vi "close buffer.vi"(8 "error in (no error)":errorcluster, 11 "Data Buffer in":refnum<class "Data Buffer.lvclass">) -> (0 "error out":errorcluster, 3 "Data Buffer out":refnum<class "Data Buffer.lvclass">)   [LabVIEW 2022 SP3, in "Data Buffer.lvclass"]
uses:
  Data Buffer.lvclass
  Data Buffer.lvclass/Data Buffer.ctl
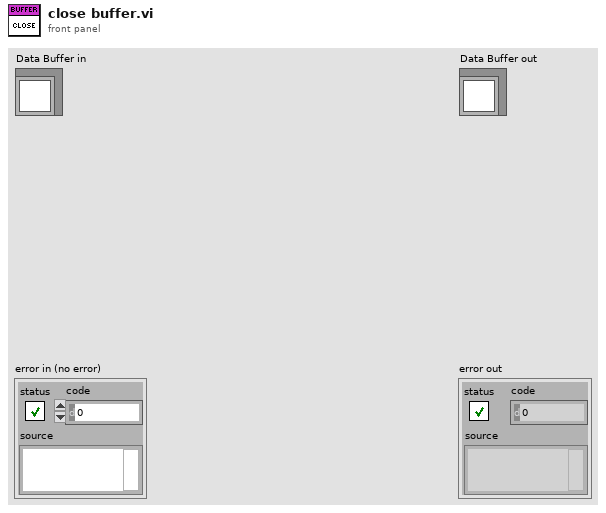
[diagram p1: front panel]
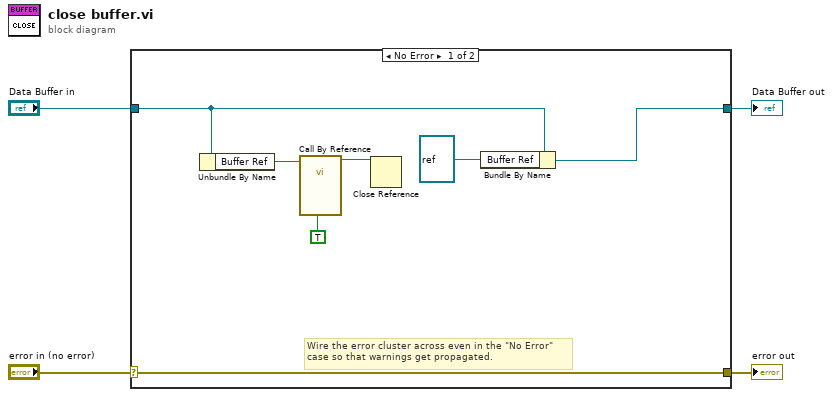
[diagram p0: block diagram]
diagram:
  n1 = case shown="No Error" "error in (no error)" {
    selector: "error in (no error)" -> [w11 w13]
    tunnel: [w11 w13] -> w3
    tunnel: [w6 w12] -> w1
    tunnel: "Data Buffer in" -> [w5 w12]
    frame No Error {
      # "Wire the error cluster across even in the \"No Error\"\ncase so that warnings get propagated."
      n2 = Unbundle By Name(w5) -> ("Buffer Ref"=w10:refnum<vi>)
      n3 = call-by-ref "?"(reference=w10, "Clear"=TRUE) -> (reference out=w8:refnum<vi>)  [unwired: 10 in, 3 out]
      n4 = Close Reference(reference=w8) -> ()  [unwired: 1 in, 1 out]
      n5 = Bundle By Name(cluster=w5, "Buffer Ref"=refnum<vi> refnum) -> (w6:refnum<class "Data Buffer.lvclass">)
    }
    frame Error {
    }
  }
  "error out" <- w3
  "Data Buffer out" <- w1
